vi "1_Celsius_To_Fahrenheit(Training).vi"() -> ()   [LabVIEW 2020]
uses:
  <vilib>/Ngene/DeepLTK/Toolkit/NN_Train/Controls/NN_Train_Params.ctl
  <vilib>/Ngene/DeepLTK/Toolkit/NN_Train/Controls/NN_Train_Optimizer.ctl
  <vilib>/Ngene/DeepLTK/Toolkit/NN_Train/Controls/NN_Train_Data_Sampling.ctl
  <vilib>/Ngene/DeepLTK/Toolkit/NN_Train/Controls/NN_LR_Policy_Cfg.ctl
  <vilib>/Ngene/DeepLTK/Toolkit/NN_Train/Controls/NN_LR_Policy_Type.ctl
  <vilib>/Ngene/DeepLTK/Toolkit/NN_Train/Controls/NN_Train_Session_Data.ctl
  <vilib>/Ngene/DeepLTK/Toolkit/NN_Data/API/DataSet_Types/NN_DataSet(In1D_Out1D).ctl
  <vilib>/Ngene/DeepLTK/Toolkit/NN_Data/API/DataRef_Types/NN_Data_ref(2D_SGL).ctl
  <vilib>/Ngene/DeepLTK/Toolkit/NN_Data/API/DataRef_Types/NN_Data_ref(1D_I32).ctl
  <vilib>/Ngene/DeepLTK/Toolkit/NN_Layers/Layers/Input/Controls/NN_Layer_Config(Input1D).ctl
  <vilib>/Ngene/DeepLTK/Toolkit/NN_Layers/Layers/FC/Controls/NN_Layer_Config(FC).ctl
  <vilib>/Ngene/DeepLTK/Toolkit/NN_Activations/Controls/NN_Activation_Type.ctl
  <vilib>/Ngene/DeepLTK/Toolkit/NN_Layers/Controls/NN_Layer_Init_Params.ctl
  <vilib>/Ngene/DeepLTK/Toolkit/NN_Layers/Controls/NN_Layer_Weight_Init_Type.ctl
  <vilib>/Ngene/DeepLTK/Toolkit/NN_Layers/Layers/Input/NN_Layer_Create(Input1D).vi
  <vilib>/Ngene/DeepLTK/Toolkit/NN_Layers/Layers/FC/NN_Layer_Create(FC).vi
  <vilib>/Ngene/DeepLTK/Toolkit/NN_Train/Loss_Functions/NN_Set_Loss(MSE).vi
  <vilib>/Ngene/DeepLTK/Toolkit/Deep_Learning_Toolkit_by_Ngene.lvlib
panel:
  out "Loss Value":sgl format="%#_3g"
  out "Session Data":T1={"Epochs"=2186.8, "Tot_Iter"=5467, "LR"=0.002, "LR_iter"=1}
  in  "Stop Training":bool
  in  "LR_Decay_Params":T2={"Policy_Type"=enum."Manual", "LR0"=0.002, "k"=0.0, "WarmUp_Policy"=enum."Step", "WarmUp_Iter"=100, "WarmUp_Ratio"=10.0} {"WarmUp_Ratio" min=1; "WarmUp_Iter" min=1; "LR0" format="%.7f"}
  out "Loss":sgl(graph)=3.7212885e-08
  in  "NN_Train_Params":T4={"Optimizer"=enum."SGD", "Beta_1"=0.9, "Beta_2"=0.0, "Weight Decay(L1)"=1e-07, "Weight Decay(L2)"=1e-07, "Data_Sampling"=enum."Sequential"}
  # "Overview: Demonstrates the usage of Deep Learning Toolkit for solving a Celius to Fahrenheit (C2F) convertion problem.\nRequirements: DeepLTK - Deep Learning Toolkit for LabVIEW (https://www.ngene.co/deep-learning-toolkit-for-labview)\nInstructions:\n1. Run the VI.\n2. Observe how the training loss is decreasing.\n3. Observe the training speed.\n4. Press the Stop Train button when the curve stops decreasing.\nMore Examples:  https://github.com/ngenehub/deepltk_examples"
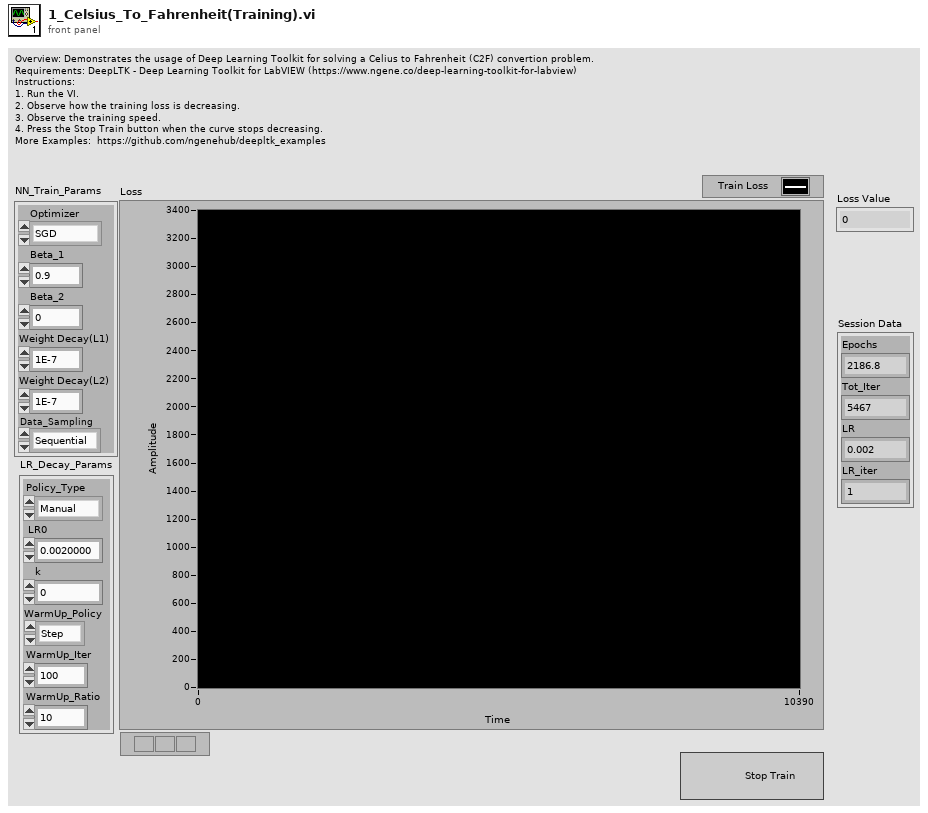
[diagram p1: front panel]
types:
  T1 = typedef "Deep_Learning_Toolkit_by_Ngene.lvlib/NN_Train_Session_Data.ctl" = cluster{"Epochs":sgl, "Tot_Iter":i32, "LR":sgl, "LR_iter":i32}
  T2 = typedef "Deep_Learning_Toolkit_by_Ngene.lvlib/NN_LR_Policy_Cfg.ctl" = cluster{"Policy_Type":T3, "LR0":dbl, "k":sgl, "WarmUp_Policy":enum16{"Step", "Ramp"}, "WarmUp_Iter":i32, "WarmUp_Ratio":sgl}
  T3 = typedef "Deep_Learning_Toolkit_by_Ngene.lvlib/NN_LR_Policy_Type.ctl" = enum16{"Manual", "Step", "Exp", "1/t"}
  T4 = typedef "Deep_Learning_Toolkit_by_Ngene.lvlib/NN_Train_Params.ctl" = cluster{"Optimizer":T5, "Beta_1":sgl, "Beta_2":sgl, "Weight Decay(L1)":sgl, "Weight Decay(L2)":sgl, "Data_Sampling":T6}
  T5 = typedef "Deep_Learning_Toolkit_by_Ngene.lvlib/NN_Train_Optimizer.ctl" = enum16{"SGD", "Adam", "Adagrad", "Adadelta", "RMSProp", "Nesterov"}
  T6 = typedef "Deep_Learning_Toolkit_by_Ngene.lvlib/NN_Train_Data_Sampling.ctl" = enum16{"Random", "Sequential"}
  T7 = typedef "Deep_Learning_Toolkit_by_Ngene.lvlib/NN_Layer_Config(FC).ctl" = cluster{"Name":string, "Size":i32, "BN":bool, "Activation":T8, "Init_Params":T9, "Custom_Params":string}
  T8 = typedef "Deep_Learning_Toolkit_by_Ngene.lvlib/NN_Activation_Type.ctl" = enum16{"Sigmoid", "ReLU", "LReLU", "ReLU6", "tanh", "Swish", "Mish", "None"}
  T9 = typedef "Deep_Learning_Toolkit_by_Ngene.lvlib/NN_Layer_Init_Params.ctl" = cluster{"Init_Type":T10, "Value":sgl}
  T10 = typedef "Deep_Learning_Toolkit_by_Ngene.lvlib/NN_Layer_Weight_Init_Type.ctl" = enum16{"Const", "Uniform", "Gaussian", "Xavier"}
  T11 = typedef "Deep_Learning_Toolkit_by_Ngene.lvlib/NN_Layer_Config(Input1D).ctl" = cluster{"Name":string, "Size":i32}
  T12 = typedef "Deep_Learning_Toolkit_by_Ngene.lvlib/NN_DataSet(In1D_Out1D).ctl" = cluster{"Inputs Ref.":T13, "Outputs Ref.":T13, "Dims_In":i32, "Dataset_Size":i32, "Outputs_idx Ref.":T14, "Dims_Out":i32, "Labels":string[], "File Paths":path[]}
  T13 = typedef "Deep_Learning_Toolkit_by_Ngene.lvlib/NN_Data_ref(2D_SGL).ctl" = refnum<data-value>
  T14 = typedef "Deep_Learning_Toolkit_by_Ngene.lvlib/NN_Data_ref(1D_I32).ctl" = refnum<data-value>
  T15 = typedef "Deep_Learning_Toolkit_by_Ngene.lvlib/NN.ctl" = cluster{"Name":string, "No of Layers":i32, "mBatch":i32, "Layers":T16[], "Dimty":T17, "Dims_In":T18, "Dims_Out":T18, "Working_Dir":path, "Train?":bool, "Train_Params":T4, "LR_Update_Policy":T2, "Session Data":T1, "Ground_truth":T19, "NNg_hdls":T20, "NN_Device":T21, "GPU Id":i32, "Labels":string[], "Receptive Field":T22[], "Loss_Type":T23, "Loss_Cfg_Prms":variant}
  T16 = typedef "Deep_Learning_Toolkit_by_Ngene.lvlib/NN_Layer_ref.ctl" = refnum<data-value>
  T17 = typedef "Deep_Learning_Toolkit_by_Ngene.lvlib/NN_In_Out_Dim-ty.ctl" = enum8{"In1D_Out1D", "In3D_Out1D", "In3D_Out3D", "In3D_OutBBox"}
  T18 = typedef "Deep_Learning_Toolkit_by_Ngene.lvlib/NN_Dims(C,H,W).ctl" = cluster{"C":i32, "H":i32, "W":i32}
  T19 = typedef "Deep_Learning_Toolkit_by_Ngene.lvlib/NN_Ground_truth.ctl" = cluster{"Y":variant, "Y_idx":T14}
  T20 = typedef "Deep_Learning_Toolkit_by_Ngene.lvlib/nng_cuda_handles.ctl" = cluster{"cudnn":u64, "cublas":u64, "stream":u64, "curand":u64}
  T21 = typedef "Deep_Learning_Toolkit_by_Ngene.lvlib/NN_Device.ctl" = enum16{"CPU", "GPU"}
  T22 = typedef "Deep_Learning_Toolkit_by_Ngene.lvlib/NN_Dims(V,H).ctl" = cluster{"V":i32, "H":i32}
  T23 = typedef "Deep_Learning_Toolkit_by_Ngene.lvlib/NN_Loss_Type.ctl" = enum16{"None", "MSE", "CrossEntropy", "YOLO_v2"}
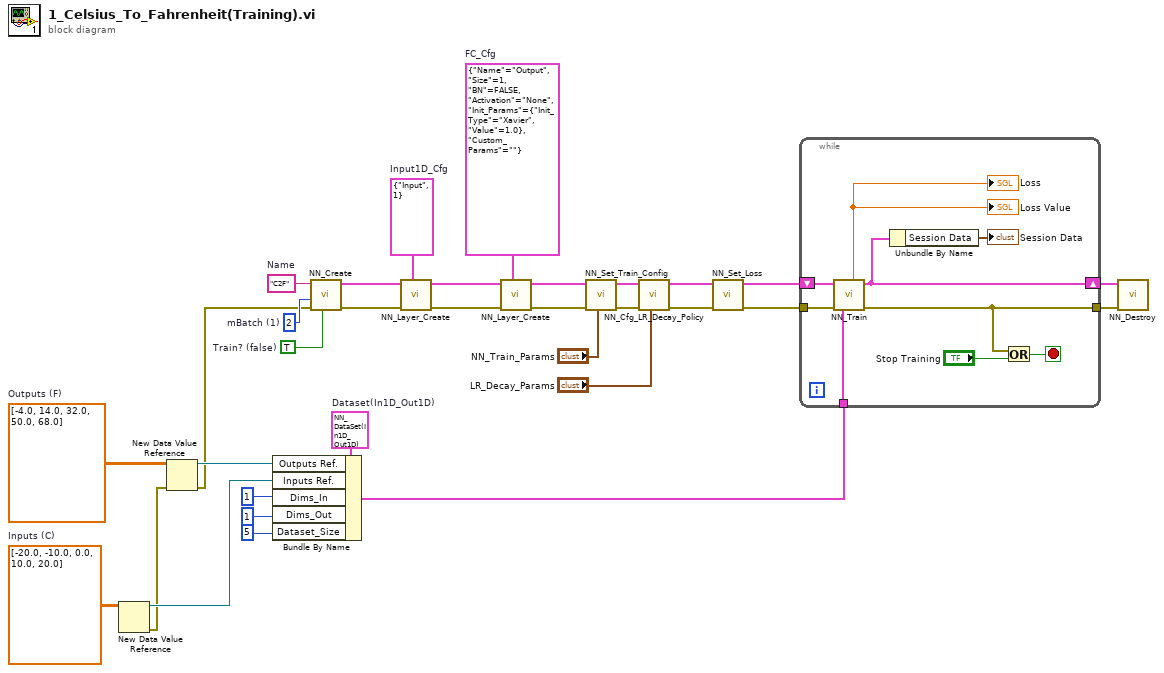
[diagram p0: block diagram]
diagram:
  w15 = 2  # mBatch (1)
  w28 = T7 {"Name"="Output", "Size"=1, "BN"=FALSE, "Activation"=enum."None", "Init_Params"={"Init_Type"=enum."Xavier", "Value"=1.0}, "Custom_Params"=""}  # FC_Cfg
  w29 = T11 {"Name"="Input", "Size"=1}  # Input1D_Cfg
  w30 = T12 {"Inputs Ref."=refnum, "Outputs Ref."=refnum, "Dims_In"=0, "Dataset_Size"=0, "Outputs_idx Ref."=refnum, "Dims_Out"=0, "Labels"=[], "File Paths"=[]}  # Dataset(In1D_Out1D)
  w31 = "C2F"  # Name
  w32 = TRUE  # Train? (false)
  w26 = sgl[][] [[-4.0], [14.0], [32.0], [50.0], [68.0]]  # Outputs (F)
  w27 = sgl[][] [[-20.0], [-10.0], [0.0], [10.0], [20.0]]  # Inputs (C)
  n1 = New Data Value Reference(data value=w27) -> (data value reference=w25:refnum<data-value>, error out=w23:errorcluster)  [unwired: 1 in]
  n2 = New Data Value Reference(data value=w26, error in=w23) -> (data value reference=w24:refnum<data-value>, error out=w9:errorcluster)
  n3 = Bundle By Name(cluster=w30, "Outputs Ref."=w24, "Inputs Ref."=w25, "Dims_In"=1, "Dims_Out"=1, "Dataset_Size"=5) -> (w4:T12)
  n4 = call <vilib>:"NN_Create.vi"("Train? (false)"=w32, "error in (no error)"=w9, "mBatch (1)"=w15, "Name"=w31) -> ("error out"=w8:errorcluster, "NN out"=w12:T15)  [unwired: 6 in]
  n5 = call-poly <vilib>:"NN_Layer_Create.vi"("Input1D_Cfg"=w29, "error in (no error)"=w8, "NN in"=w12) -> ("error out"=w7:errorcluster, "NN out"=w11:T15)  [unwired: 6 in, 1 out]
  n6 = call-poly <vilib>:"NN_Layer_Create.vi"("FC_Cfg"=w28, "error in (no error)"=w7, "NN in"=w11) -> ("error out"=w6:errorcluster, "NN out"=w10:T15)  [unwired: 6 in, 1 out]
  n7 = call <vilib>:"NN_Set_Train_Config.vi"("NN_Train_Params"="NN_Train_Params", "error in (no error)"=w6, "NN in"=w10) -> ("error out"=w20:errorcluster, "NN out"=w19:T15)  [unwired: 7 in]
  n8 = call <vilib>:"NN_Cfg_LR_Decay_Policy.vi"("LR_Decay_Params"="LR_Decay_Params", "error in (no error)"=w20, "NN in"=w19) -> ("error out"=w2:errorcluster, "NN out"=w5:T15)  [unwired: 7 in]
  n9 = call-poly <vilib>:"NN_Set_Loss.vi"("error in (no error)"=w2, "NN in"=w5) -> ("error out"=w1:errorcluster, "NN out"=w3:T15)  [unwired: 8 in]
  n10 = while {
    shift-right: [w41] -> w14
    shift-left: w3 -> [w39]
    tunnel: [w34] -> w13
    tunnel: w1 -> [w38]
    tunnel: w4 -> [w37]
    stop <- w33 stop-if-true
    n11 = call <vilib>:"NN_Train.vi"("Train Dataset"=w37, "error in (no error)"=w38, "NN in"=w39) -> ("error out"=w34:errorcluster, "NN out"=w41:T15, "Loss"=→"Loss" →"Loss Value":sgl)  [unwired: 5 in, 1 out]
    n12 = Unbundle By Name(w41) -> ("Session Data"=→"Session Data":T1)
    n13 = Or(x=w34, y="Stop Training") -> (x .or. y?=w33:bool)
  }
  n14 = call <vilib>:"NN_Destroy.vi"("error in (no error)"=w13, "NN in"=w14) -> ()  [unwired: 9 in, 1 out]
